vi "Get Power Meter Default Value.vi"(0 "SG Path PM Accessor in":refnum<class "SG Path Accessor.lvclass">, 11 "error in":errorcluster) -> (4 "SG Path PM Accessor out":refnum<class "SG Path Accessor.lvclass">, 6 "Power Meter out":refnum<class "Power Meter Base.lvclass">, 15 "error out":errorcluster)   [LabVIEW 2023, in "NI Cal-5501 Power Detector.lvlib" / "SG Path Accessor.lvclass"]
uses:
  SG Path Accessor.lvclass
  Instruments/Power Meter/Power Meter Base/Power Meter Base.lvclass
  Power Detector/Power Detector.lvclass
  C:/srd-semi-rfcal-software/AuxTools/STSRFFixtureCharactUtility/Source/Code Modules/Fixture/Instruments/Power Meter/Power Meter Base/Power Meter Base.lvclass
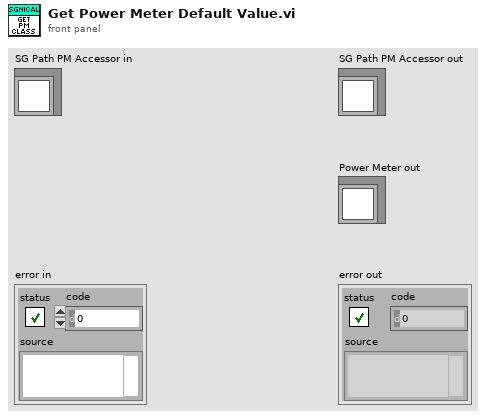
[diagram p1: front panel]
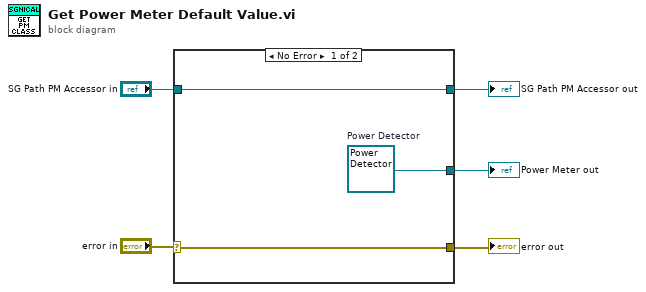
[diagram p0: block diagram]
diagram:
  n1 = case shown="No Error" "error in" {
    selector: "error in" -> [w7 w9]
    tunnel: "SG Path PM Accessor in" -> [w8 w10]
    tunnel: [w8 w10] -> w5
    tunnel: [w7 w9] -> w2
    tunnel: [w6 _] -> w4
    frame No Error {
      w6 = refnum<class "Power Detector.lvclass"> refnum  # Power Detector
    }
    frame Error {
    }
  }
  "error out" <- w2
  "SG Path PM Accessor out" <- w5
  "Power Meter out" <- w4
